vi "String to 1D Array_csm.vi"(5 "ignore duplicate delimiters? (F=No)":bool, 7 "delimiter (Tab)":string="\t", 10 "string":string) -> (1 "Array of Strings":string[](array[string]))   [LabVIEW 2020, in "Communicable State Machine.lvlib"]
doc: "Converts delimited string to a 1D array."
uses:
  Communicable State Machine.lvlib
panel:
  # "[OpenG VI Tags] ***Do Not Remove***"
  # "d"
  # "String to 1D Array.vi\n\nConverts delimited string to a 1D array.\n\nPlease visit http://www.OpenG.org to learn about the\nOpen Source LabVIEW software movement.\n\nNOTICE -- YOU MUST LEAVE THIS NOTICE IN PLACE.  PER THE TERMS OF THE LICENSE BELOW, YOU MAY SUBLICENSE THIS SOFTWARE \nIN ANY WAY THAT DOES NOT CONFLICT WITH THIS LICENSE.\n\n### BSD License (http://www.opensource.org/licenses/bsd-license.php) Begin ###\n \nCopyright (c) 2002, Jim Kring <jim@jimkring.com>\nCopyright (c) 2005, MKS Instruments, Inc., author: Doug Femec<doug_femec@mksinst.com>, IM dafemec\n\nAll rights reserved.\n\nRedistribution and use in source and binary forms, with or without modification, are permitted provided that the following conditions are met:\n\n    * Redistributions of source code must retain the above copyright notice, this list of conditions and the following disclaimer.\n    * Redistributions in binary form must reproduce the above copyright notice, this list of conditions and the following disclaimer in the \n       documentation and/or other materials provided with the distribution.\n    * Neither the name of SciWare, James Kring, Inc., nor the names of its contributors may be used to endorse or promote products derived \n       from this software without specific prior written permission.\n\nTHIS SOFTWARE IS PROVIDED BY THE COPYRIGHT HOLDERS AND CONTRIBUTORS \"AS IS\" AND ANY EXPRESS OR IMPLIED WARRANTIES, \nINCLUDING, BUT NOT LIMITED TO, THE IMPLIED WARRANTIES OF MERCHANTABILITY AND FITNESS FOR A PARTICULAR PURPOSE ARE \nDISCLAIMED. IN NO EVENT SHALL THE COPYRIGHT OWNER OR CONTRIBUTORS BE LIABLE FOR ANY DIRECT, INDIRECT, INCIDENTAL,\n SPECIAL, EXEMPLARY, OR CONSEQUENTIAL DAMAGES (INCLUDING, BUT NOT LIMITED TO, PROCUREMENT OF SUBSTITUTE GOODS OR \nSERVICES; LOSS OF USE, DATA, OR PROFITS; OR BUSINESS INTERRUPTION) HOWEVER CAUSED AND ON ANY THEORY OF LIABILITY, \nWHETHER IN CONTRACT, STRICT LIABILITY, OR TORT (INCLUDING NEGLIGENCE OR OTHERWISE) ARISING IN ANY WAY OUT OF THE USE \nOF THIS SOFTWARE, EVEN IF ADVISED OF THE POSSIBILITY OF SUCH DAMAGE.\n\n### BSD License End ###"
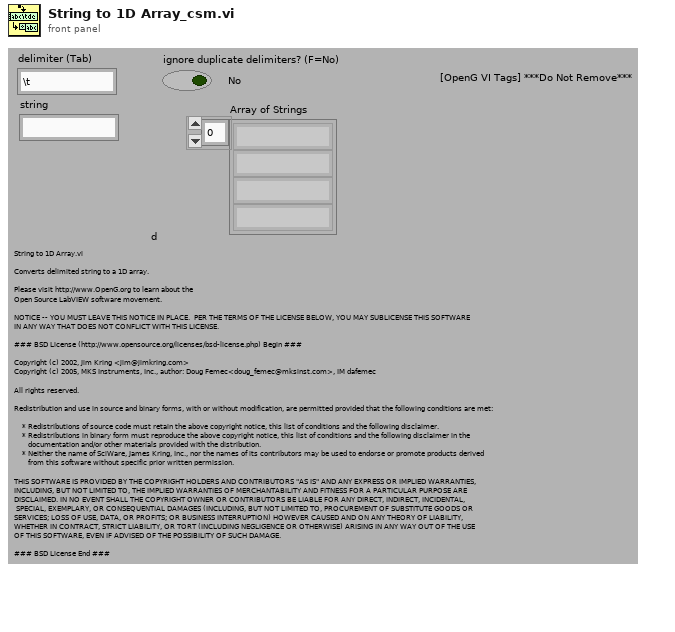
[diagram p1: front panel]
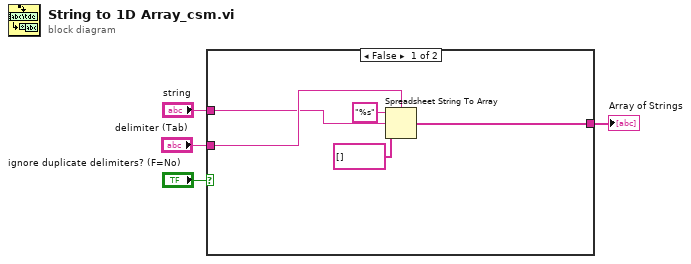
[diagram p0: block diagram]
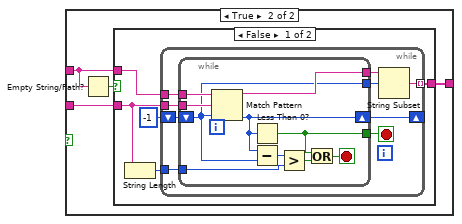
[diagram p2: hidden frame]
diagram:
  n1 = case shown="False" "ignore duplicate delimiters? (F=No)" {
    tunnel: "string" -> [w5 w11]
    tunnel: [w7 w13] -> w1
    tunnel: "delimiter (Tab)" -> [w6 w12]
    frame False {
      n2 = Spreadsheet String To Array(delimiter (Tab)=w6, format string="%s", spreadsheet string=w5, array type (2D Dbl)=string[] [] ("Array of Strings")) -> (array=w7:string[])
    }
    frame True {
      n3 = Empty String/Path?(string/path=w11) -> (empty?=w10:bool)
      n4 = case shown="False" w10 {
        tunnel: w11 -> [w18 _]
        tunnel: [w16 _] -> w13
        tunnel: w12 -> [w15 _]
        frame False {
          n5 = String Length(string=w15) -> (length=w14:i32)
          n6 = while {
            shift-right: [w22] -> _
            shift-left: -1 -> [w20]
            tunnel: w18 -> [w27]
            tunnel: w15 -> [w26]
            tunnel: [w25] -> w16 mode=indexing
            tunnel: w14 -> [w24]
            stop <- w23 stop-if-true
            n7 = while {
              tunnel: w27 -> [w37]
              tunnel: w26 -> [w36]
              tunnel: w24 -> [w34]
              tunnel: [w33] -> w23
              shift-right: [w31] -> w22
              shift-left: w20 -> [w29]
              tunnel: [w30] -> w21
              tunnel: [w29] -> w19
              stop <- w32 stop-if-true
              n8 = Match Pattern(string=w37, regular expression=w36, offset (0)=w29) -> (before substring=w30:string, offset past match=w31:i32)  [unwired: 2 out]
              n9 = Less Than 0?(x=w31) -> (x < 0?=w33:bool)
              n10 = Subtract(x=w31, y=w29) -> (x-y=w35:i32)
              n11 = Greater?(x=w35, y=w34) -> (0:w28:bool)
              n12 = Or(x=w33, y=w28) -> (x .or. y?=w32:bool)
            }
            n13 = String Subset(string=w21, offset (0)=w19) -> (substring=w25:string)  [unwired: 1 in]
          }
        }
        frame True {
        }
      }
    }
  }
  "Array of Strings" <- w1
